vi "Close Component UI.vi"(10 "output cluster":T1, 11 "Gantry In":refnum<k24>) -> (3 "Gantry Out":refnum<k24>)   [LabVIEW 2021, in "Component Tray.lvclass"]
uses:
  Component Tray.lvclass
  C:/Program Files (x86)/Aerotech/A3200/LabVIEW/2010/Bin/Aerotech.A3200.dll
  Program Files (x86)/Aerotech/A3200/LabVIEW/2010/Bin/Aerotech.A3200.dll
  Find Component.ctl
  Controller/Camera/Machine Vision.ctl
  Component Tray.lvclass/Component Tray.ctl
  Controller/Motion/A3200/A3200.lvclass
  Controller/Camera/Camera.lvclass
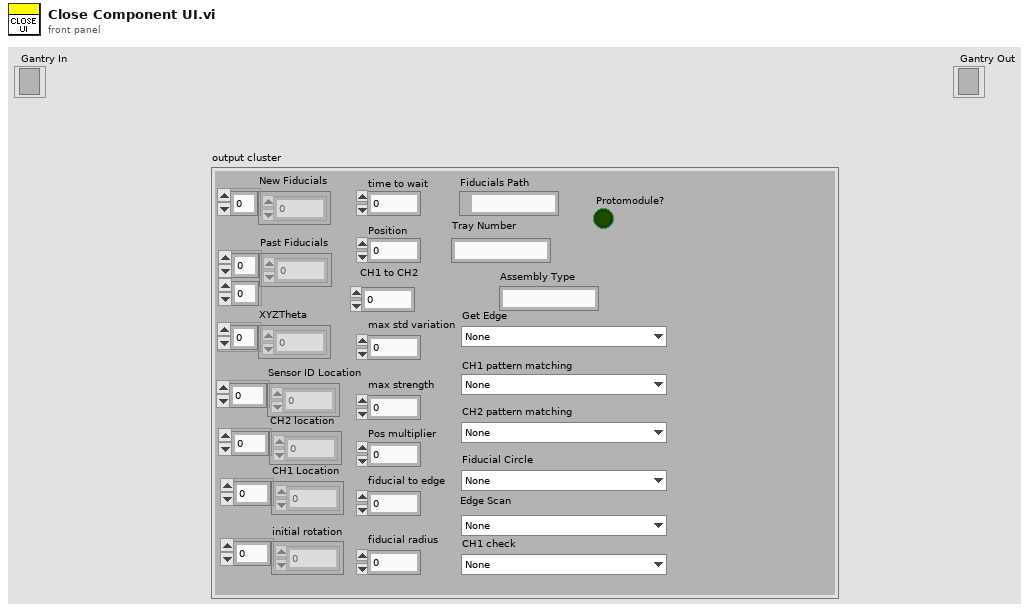
[diagram p1: front panel]
types:
  T1 = typedef "Component Tray.lvclass/Find Component.ctl" = cluster{"New Fiducials":dbl[], "Past Fiducials":dbl[][], "XYZTheta":dbl[], "Fiducials Path":path, "Position":i32, "CH1 Location":dbl[], "Sensor ID Location":dbl[], "initial rotation":dbl[], "CH2 location":dbl[], "max std variation":dbl, "max strength":dbl, "CH2 pattern matching":T2, "Fiducial Circle":T2, "Get Edge":T2, "Pos multiplier":dbl, "time to wait":u32, "fiducial to edge":dbl, "Protomodule?":bool, "Assembly Type":string, "CH1 to CH2":dbl, "Tray Number":string, "fiducial radius":dbl, "4 fiducials?":bool, "CH1 check":T2, "Edge Scan":T2, "CH1 pattern matching":T2, "Sensor Thickness":dbl}
  T2 = typedef "Camera.lvclass/Machine Vision.ctl" = enum16{"None", "Assembly Tray Circle", "Assembly Tray Fiducial", "Partial Hexaboard", "sensor edge init", "HB edge init", "sensor edge pos1", "sensor edge pos2", "HB edge pos1", "HB edge pos2", "Sensor CH1-2", "HB CH1", "HB CH2", "V3 Sensor Circle", "Hexaboard Circle", "sensor CH1 check", "HB CH1 check "}
  T3 = typedef "File Paths.ctl" = cluster{"Glue Pattern Folder":path, "Carrier Tray Folder":path, "Pick Up Tool Fixture Folder":path, "Components Folder":path, "Bellows Tool Offset.txt":path, "Pick Up Tool Offset.txt":path, "Dispense Tip Offset.txt":path, "Log Files":path, "Gantry Assembly Map.txt":path, "Syringe and offset map.txt":path, "Controllers Folder":path, "Local dbase config":path}
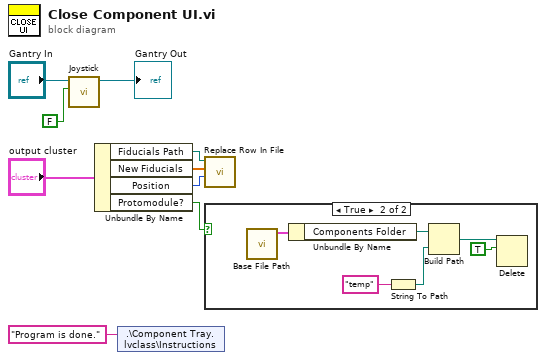
[diagram p0: block diagram]
diagram:
  n1 = call "Joystick.vi"("Joystick"=FALSE, "Gantry In"="Gantry In") -> ("Gantry Out"=→"Gantry Out":refnum<k24>)  [unwired: 8 in, 1 out]
  n2 = Unbundle By Name("output cluster") -> ("Fiducials Path"=w6:path, "New Fiducials"=w5:dbl[], "Position"=w4:i32, "Protomodule?"=w1:bool)
  n3 = shared-variable ".\\Component Tray.lvclass\\Instructions"("Program is done." ("Instructions")) -> ()  [unwired: 1 in, 1 out]
  n4 = call "Replace Row In File.vi"("Index"=w4, "Insert Array"=w5, "Path"=w6) -> ()  [unwired: 8 in, 1 out]
  n5 = case shown="True" w1 {
    frame False {
    }
    frame True {
      n6 = call "Base File Path.vi"() -> ("Paths Out"=w14:T3)  [unwired: 11 in]
      n7 = Unbundle By Name(w14) -> ("Components Folder"=w12:path)
      n8 = String To Path(string="temp") -> (path=w13:path)
      n9 = Build Path(base path=w12, name or relative path=w13) -> (appended path=w15:path)
      n10 = Delete(path (use dialog)=w15, entire hierarchy (F)=TRUE) -> ()  [unwired: 3 in, 3 out]
    }
  }
